vi "F Dwf Analog Out Node Data Info.vi"(6 "pnSamplesMax":i32, 7 "pnSamplesMin":i32, 8 "error in (no error)":errorcluster, 9 "node":i32, 10 "idxChannel":i32, 11 "hdwf":i32) -> (0 "error out":errorcluster, 3 "function return":i32, 4 "pnSamplesMax out":i32, 5 "pnSamplesMin out":i32)   [LabVIEW 2019, in "Olasdwf.lvlib"]
doc: "DWFAPI int FDwfAnalogOutNodeDataInfo(HDWF hdwf, int idxChannel, AnalogOutNode node, int *pnSamplesMin, int *pnSamplesMax);"
uses:
  Olasdwf.lvlib
  Windows/System32/dwf.dll
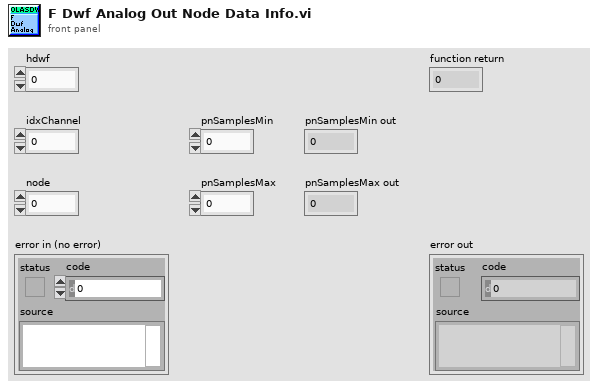
[diagram p1: front panel]
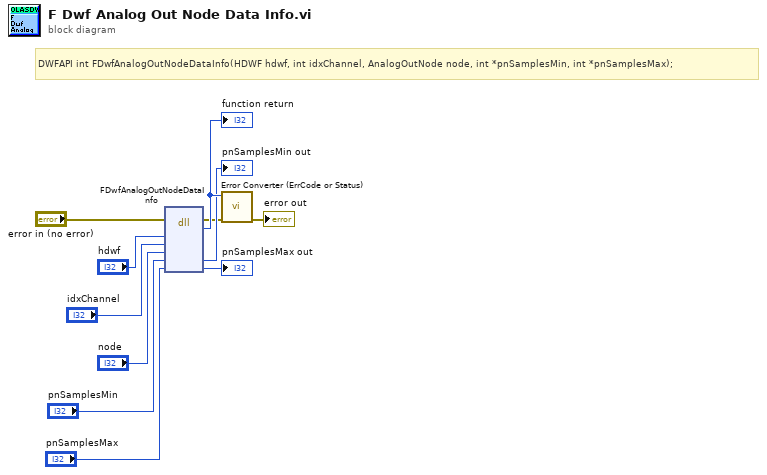
[diagram p0: block diagram]
diagram:
  # "DWFAPI int FDwfAnalogOutNodeDataInfo(HDWF hdwf, int idxChannel, AnalogOutNode node, int *pnSamplesMin, int *pnSamplesMax);"
  n1 = dll-call lib="C:/Windows/System32/dwf.*" fn="FDwfAnalogOutNodeDataInfo"(error in="error in (no error)", "hdwf"="hdwf", "idxChannel"="idxChannel", "node"="node", "pnSamplesMin"="pnSamplesMin", "pnSamplesMax"="pnSamplesMax") -> (error out=w2:errorcluster, w11:i32, "pnSamplesMin"=→"pnSamplesMin out":i32, "pnSamplesMax"=→"pnSamplesMax out":i32)  [unwired: 5 in, 1 out]
  "function return" <- w11
  n2 = call "Error Converter (ErrCode or Status).vi"("error in (no error)"=w2, "error code"=w11) -> ("error out"=→"error out":errorcluster)  [unwired: 9 in]
